vi "Send Dialog.vi"() -> ()   [LabVIEW 2011, in "CAN FD.lvlib"]
uses:
  CAN FD.lvlib
  Typedef/Send Data.ctl
  data_type/ZCAN_Transmit_Data.ctl
  data_type/ZCAN_TransmitFD_Data.ctl
panel:
  in  "Clear":bool
  in  "Data+":bool caption="数据递增"
  in  "ID+":bool caption="ID递增"
  in  "Stop":bool
  out "Count":u32 caption="发送统计" min=1 max=10000
  in  "Send":bool
  in  "spare":u32=100 caption="发送间隔(ms)" max=10000
  in  "Frames":u32=1 caption="单次帧数" min=1 max=1000
  in  "Times":i32=1 caption="发送次数(-1=持续)" min=-1
  in  "Data":string="01 23 45 67 89 AB CD EF" caption="数据输入"
  in  "Len":u8(ring)=8 caption="数据长度" items=["0"=0, "1"=1, "2"=2, "3"=3, "4"=4, "5"=5, "6"=6, "7"=7, "8"=8, "12"=12, "16"=16, "20"=20, "24"=24, "32"=32, "48"=48, "64"=64]
  in  "ID":u32=256 max=2047 format="0x%03x"
  in  "FD":u8(ring) caption="CANFD加速" items=["不加速", "加速"]
  in  "Protocol":u32(ring) caption="协议" items=["CAN", "CANFD"]
  in  "Type":u32(ring) caption="帧格式" items=["标准帧", "扩展帧"]
  in  "Format":u32(ring) caption="帧格式" items=["数据帧", "远程帧"]
  in  "Mode":u32(ring) caption="发送方式" items=["正常发送", "单次发送", "自发自收", "单次自发自收"]
  in  "Channel":u32(ring) caption="通道选择" items=["USBCANFD-200U 设备0 通道0"=2686976, "USBCANFD-200U 设备0 通道1"=2686977]
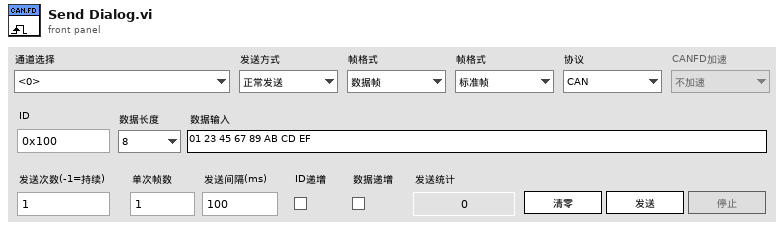
[diagram p1: front panel]
types:
  T1 = typedef "CAN FD.lvlib/Send Data.ctl" = cluster{"Handle":u32, "Frames":u32, "Spare":u32, "Times":i32, "ID+":bool, "Data+":bool, "Type":enum16{"CAN", "CANFD"}, "Data":variant}
  T2 = typedef "ZCAN_Transmit_Data.ctl" = cluster{"帧类型":u32, "帧格式":u32, "ID":u32, "数据长度":u8, "DATA":cluster{"CAN数据[0]":u8, "CAN数据[1]":u8, "CAN数据[2]":u8, "CAN数据[3]":u8, "CAN数据[4]":u8, "CAN数据[5]":u8, "CAN数据[6]":u8, "CAN数据[7]":u8}, "发送方式":u32}
  T3 = typedef "ZCAN_TransmitFD_Data.ctl" = cluster{"帧类型":u32, "帧格式":u32, "ID":u32, "数据长度":u8, "CANFD加速？":u8, "DATA":cluster{"CAN数据[0]":u8, "CAN数据[1]":u8, "CAN数据[2]":u8, "CAN数据[3]":u8, "CAN数据[4]":u8, "CAN数据[5]":u8, "CAN数据[6]":u8, "CAN数据[7]":u8, "CAN数据[8]":u8, "CAN数据[9]":u8, "CAN数据[10]":u8, "CAN数据[11] ":u8, "CAN数据[12] ":u8, "CAN数据[13] ":u8, "CAN数据[14] ":u8, "CAN数据[15] ":u8, "CAN数据[16]":u8, "CAN数据[17]":u8, "CAN数据[18]":u8, "CAN数据[19]":u8, "CAN数据[20]":u8, "CAN数据[21]":u8, "CAN数据[22]":u8, "CAN数据[23]":u8, "CAN数据[24] ":u8, "CAN数据[25]":u8, "CAN数据[26]":u8, "CAN数据[27]":u8, "CAN数据[28]":u8, "CAN数据[29]":u8, "CAN数据[30]":u8, "CAN数据[31]":u8, "CAN数据[32]":u8, "CAN数据[33]":u8, "CAN数据[34]":u8, "CAN数据[35]":u8, "CAN数据[36]":u8, "CAN数据[37]":u8, "CAN数据[38]":u8, "CAN数据[39]":u8, "CAN数据[40]":u8, "CAN数据[41]":u8, "CAN数据[42]":u8, "CAN数据[43]":u8, "CAN数据[44]":u8, "CAN数据[45]":u8, "CAN数据[46]":u8, "CAN数据[47]":u8, "CAN数据[48]":u8, "CAN数据[49]":u8, "CAN数据[50]":u8, "CAN数据[51]":u8, "CAN数据[52]":u8, "CAN数据[53]":u8, "CAN数据[54]":u8, "CAN数据[55]":u8, "CAN数据[56]":u8, "CAN数据[57]":u8, "CAN数据[58]":u8, "CAN数据[59]":u8, "CAN数据[60]":u8, "CAN数据[61]":u8, "CAN数据[62]":u8, "CAN数据[63]":u8}, "发送方式":u32}
  T4 = cluster{"Data[0]":u8, "Data[1]":u8, "Data[2]":u8, "Data[3]":u8, "Data[4]":u8, "Data[5]":u8, "Data[6]":u8, "Data[7]":u8}
  T5 = cluster{"Data[0]":u8, "Data[1]":u8, "Data[2]":u8, "Data[3]":u8, "Data[4]":u8, "Data[5]":u8, "Data[6]":u8, "Data[7]":u8, "Data[8]":u8, "Data[9]":u8, "Data[10]":u8, "Data[11]":u8, "Data[12]":u8, "Data[13]":u8, "Data[14]":u8, "Data[15]":u8, "Data[16]":u8, "Data[17]":u8, "Data[18]":u8, "Data[19]":u8, "Data[20]":u8, "Data[21]":u8, "Data[22]":u8, "Data[23]":u8, "Data[24]":u8, "Data[25]":u8, "Data[26]":u8, "Data[27]":u8, "Data[28]":u8, "Data[29]":u8, "Data[30]":u8, "Data[31]":u8, "Data[32]":u8, "Data[33]":u8, "Data[34]":u8, "Data[35]":u8, "Data[36]":u8, "Data[37]":u8, "Data[38]":u8, "Data[39]":u8, "Data[40]":u8, "Data[41]":u8, "Data[42]":u8, "Data[43]":u8, "Data[44]":u8, "Data[45]":u8, "Data[46]":u8, "Data[47]":u8, "Data[48]":u8, "Data[49]":u8, "Data[50]":u8, "Data[51]":u8, "Data[52]":u8, "Data[53]":u8, "Data[54]":u8, "Data[55]":u8, "Data[56]":u8, "Data[57]":u8, "Data[58]":u8, "Data[59]":u8, "Data[60]":u8, "Data[61]":u8, "Data[62]":u8, "Data[63]":u8}
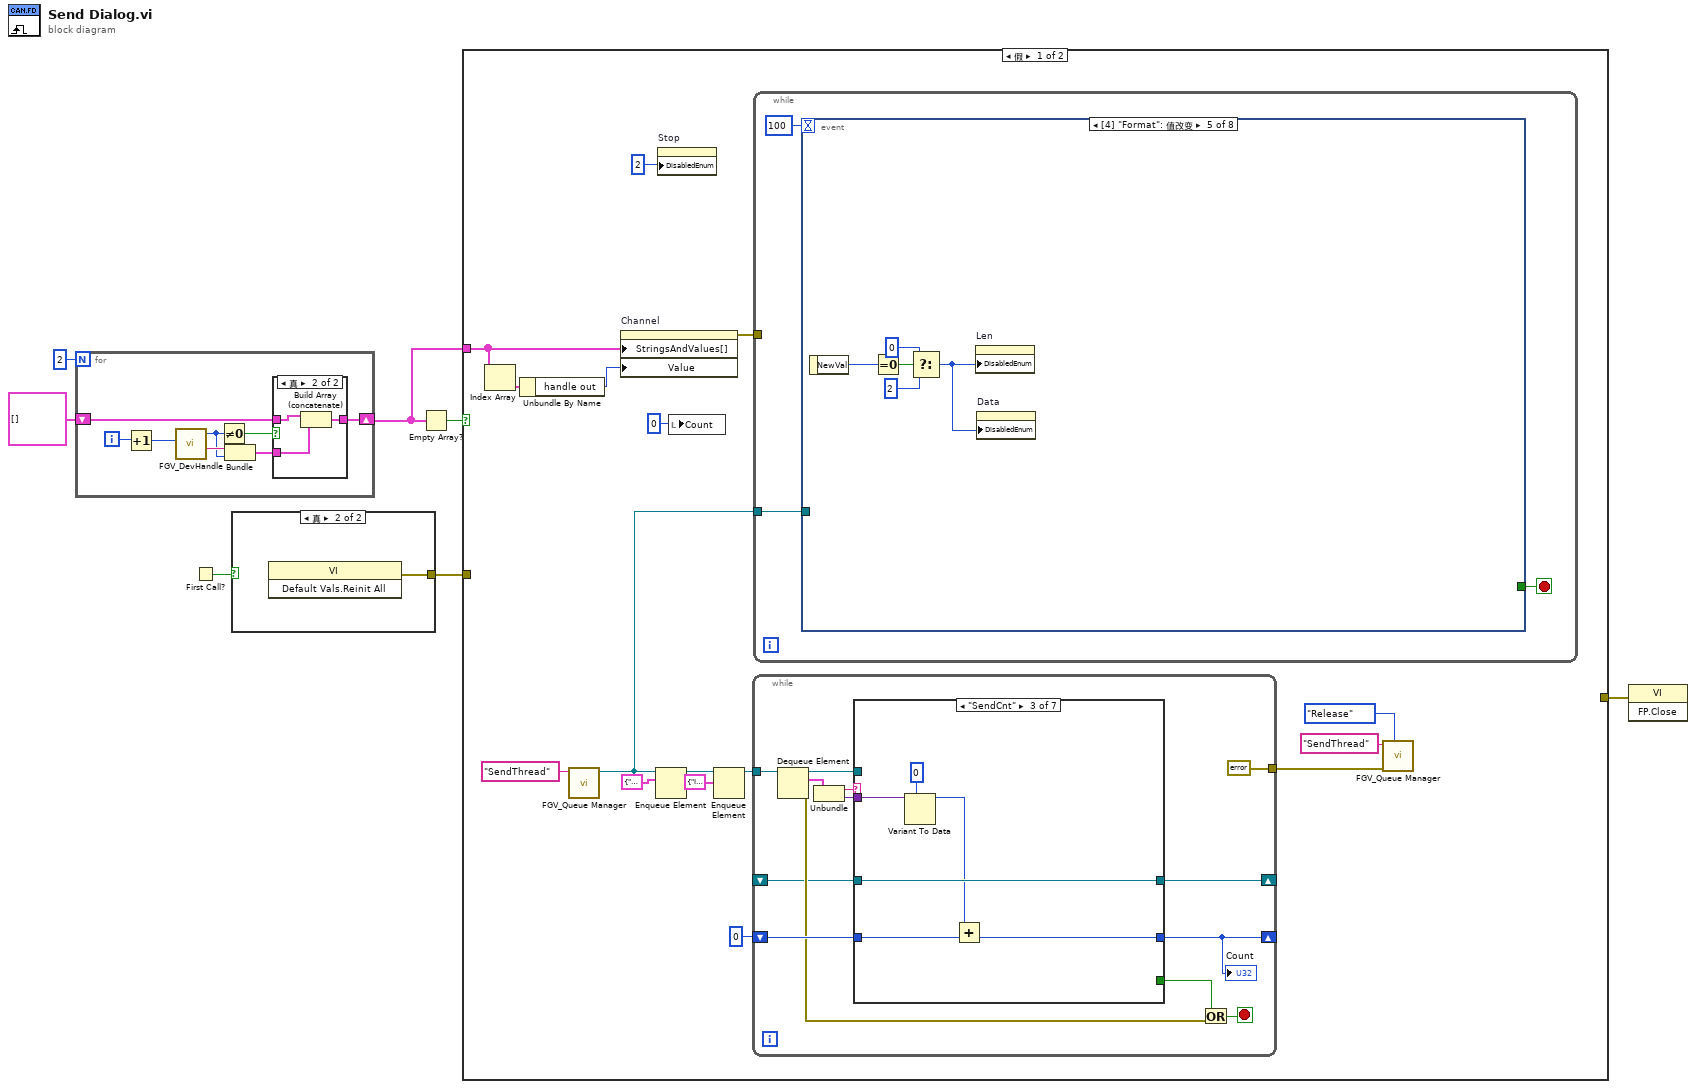
[diagram p0: block diagram]
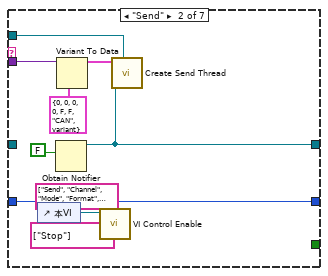
[diagram p4: hidden frame]
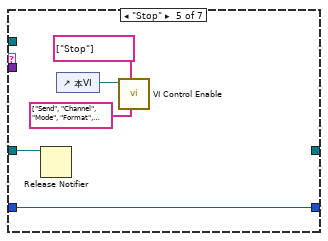
[diagram p6: hidden frame]
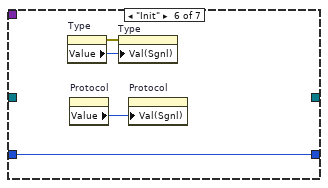
[diagram p7: hidden frame]
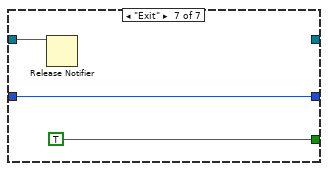
[diagram p8: hidden frame]
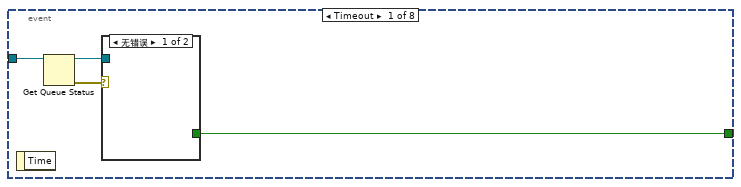
[diagram p9: hidden frame]
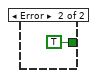
[diagram p10: hidden frame]
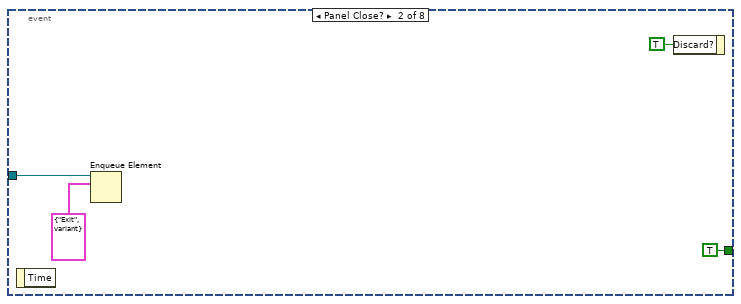
[diagram p11: hidden frame]
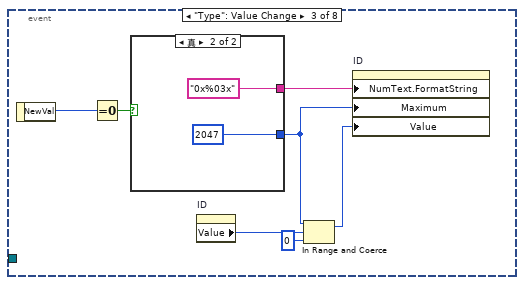
[diagram p12: hidden frame]
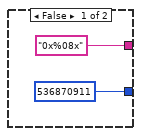
[diagram p13: hidden frame]
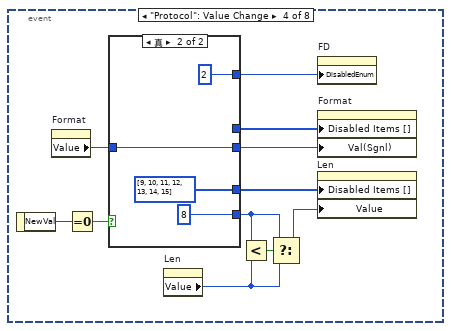
[diagram p14: hidden frame]
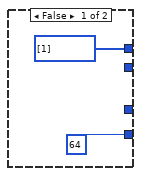
[diagram p15: hidden frame]
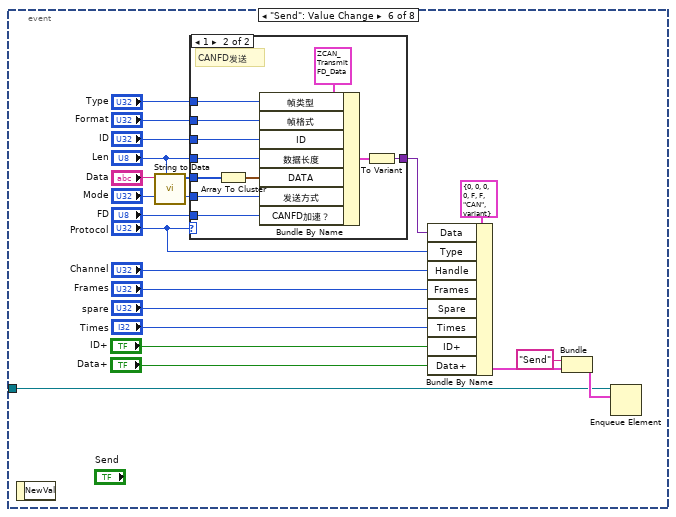
[diagram p16: hidden frame]
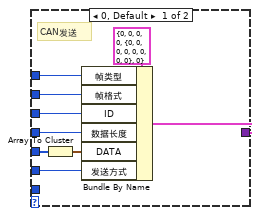
[diagram p17: hidden frame]
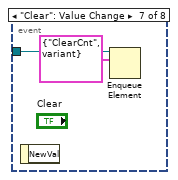
[diagram p18: hidden frame]
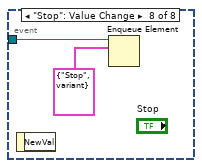
[diagram p19: hidden frame]
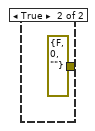
[diagram p20: hidden frame]
diagram:
  n1 = for {
    N: 2 -> [_]
    shift-right: [w9] -> w5
    shift-left: cluster{"Name out":string, "handle out":u32}[] [] -> [w8]
    i -> [w15]
    n2 = Increment(x=w15) -> (x+1=w14:i32)
    n3 = call "FGV_DevHandle.vi"("Type"=w14) -> ("Name out"=w13:string, "handle out"=w12:u32)  [unwired: 8 in, 1 out]
    n4 = Not Equal To 0?(x=w12) -> (x != 0?=w11:bool)
    n5 = Bundle("Name out"=w13, "handle out"=w12) -> (w10:cluster{"Name out":string, "handle out":u32})  [unwired: 1 in]
    n6 = case shown="真" w11 {
      tunnel: w10 -> [_ w19]
      tunnel: [w16 w18] -> w9
      tunnel: w8 -> [w16 w17]
      frame False {
      }
      frame True {
        n7 = Build Array (concatenate)(w17, w19) -> (w18:cluster{"Name out":string, "handle out":u32}[])
      }
    }
  }
  n8 = First Call?() -> (First Call?: T/F=w3:bool)
  n9 = case shown="真" w3 {
    tunnel: [_ w20] -> w2
    frame False {
    }
    frame True {
      n10 = invoke class="VI" method="Default Vals.Reinit All"() -> (error out=w20:errorcluster)  [unwired: 3 in, 2 out]
    }
  }
  n11 = Empty Array?(array=w5) -> (empty?=w4:bool)
  n12 = case shown="假" w4 {
    tunnel: w5 -> [w36 _]
    tunnel: w2 -> [_ _]
    tunnel: [_ errorcluster {"status"=FALSE, "code"=0, "source"=""} ("error constant")] -> w1
    frame False {
      n13 = Index Array(array=w36) -> (element=w35:cluster{"Name out":string, "handle out":u32})  [unwired: 1 in]
      n14 = Unbundle By Name(w35) -> ("handle out"=w34:u32)
      n15 = call "FGV_Queue Manager.vi"("Name"="SendThread") -> ("Queue"=w27:refnum<queue>)  [unwired: 8 in, 2 out]
      n16 = property on="Channel" class="Ring (严格)"("StringsAndValues[]"=w36, "Value"=w34) -> (error out=w33:errorcluster)  [unwired: 2 in, 1 out]
      n17 = Enqueue Element(queue=w27, element=cluster{"ID":string, "Data":variant} {"ID"="Stop", "Data"=variant} ("元素")) -> (queue out=w23:refnum<queue>)  [unwired: 2 in, 2 out]
      n18 = property on="Stop" class="Bool"("DisabledEnum"=2) -> ()  [unwired: 2 in, 2 out]
      n19 = local write "Count"(u32 0 ("Count")) -> ()
      n20 = Enqueue Element(queue=w23, element=cluster{"ID":string, "Data":variant} {"ID"="Init", "Data"=variant} ("元素")) -> (queue out=w22:refnum<queue>)  [unwired: 2 in, 2 out]
      n21 = while {
        tunnel: w22 -> [w49]
        shift-right: [w44] -> _
        shift-left: u32 0 -> [w45]
        tunnel: [errorcluster {"status"=FALSE, "code"=0, "source"=""} ("error constant")] -> w26
        shift-right: [w38] -> _
        shift-left: _ -> [w37]
        stop <- w39 stop-if-true
        n22 = Dequeue Element(queue=w49) -> (queue out=w43:refnum<queue>, element=w48:cluster{"ID":string, "Data":variant}, error out=w40:errorcluster)  [unwired: 2 in, 1 out]
        n23 = Unbundle(w48) -> ("ID"=w47:string, "Data"=w46:variant)
        n24 = case shown="\"SendCnt\"" w47 {
          tunnel: w46 -> [_ w60 w65 _ _ _ _]
          tunnel: [_ _ _ _ _ _ TRUE] -> w41
          tunnel: w45 -> [w50 w51 w63 _ w72 w76 w78]
          tunnel: [w50 w51 w61 _ w72 w76 w78] -> w44
          tunnel: w43 -> [_ w56 _ _ _ _ _]
          tunnel: [_ w55 w66 w67 _ _ _] -> w38
          tunnel: w37 -> [_ _ w66 w67 w68 _ w77]
          frame Default {
          }
          frame "Send" {
            n25 = control-ref of="本VI"() -> (w52:refnum<vi>)
            n26 = Obtain Notifier(notification data type=FALSE) -> (notifier out=w55:refnum<notifier>)  [unwired: 3 in, 2 out]
            n27 = Variant To Data(type=T1 {"Handle"=0, "Frames"=0, "Spare"=0, "Times"=0, "ID+"=FALSE, "Data+"=FALSE, "Type"=enum."CAN", "Data"=variant} ("Send Data"), Variant=w60) -> (data=w57:T1)  [unwired: 1 in, 1 out]
            n28 = call "VI Control Enable.vi"("Enable List"=string[] ["Stop"], "Disable List"=string[] ["Send", "Channel", "Mode", "Format", "Type", "Protocol", "FD", "ID", "Len", "Data", "Times", "Frames", "spare", "ID+", "Data+"], "VI引用句柄"=w52) -> ()  [unwired: 9 in]
            n29 = call "Create Send Thread.vi"("SendQueue"=w56, "StopNotifier"=w55, "Send Data"=w57) -> ()  [unwired: 9 in]
          }
          frame "SendCnt" {
            n30 = Variant To Data(type=u32 0, Variant=w65) -> (data=w62:u32)  [unwired: 1 in, 1 out]
            n31 = Add(x=w62, y=w63) -> (x+y=w61:u32)
          }
          frame "ClearCnt" {
          }
          frame "Stop" {
            n32 = Release Notifier(notifier=w68) -> ()  [unwired: 2 in, 3 out]
            n33 = control-ref of="本VI"() -> (w71:refnum<vi>)
            n34 = call "VI Control Enable.vi"("Enable List"=string[] ["Send", "Channel", "Mode", "Format", "Type", "Protocol", "FD", "ID", "Len", "Data", "Times", "Frames", "spare", "ID+", "Data+"] ("Disable List"), "Disable List"=string[] ["Stop"] ("Enable List"), "VI引用句柄"=w71) -> ()  [unwired: 9 in]
          }
          frame "Init" {
            n35 = property on="Type" class="Ring (严格)"() -> (error out=w74:errorcluster, "Value"=w73:u32)  [unwired: 2 in, 1 out]
            n36 = property on="Protocol" class="Ring (严格)"() -> ("Value"=w75:u32)  [unwired: 2 in, 2 out]
            n37 = property on="Type" class="Ring (严格)"(error in=w74, "Val(Sgnl)"=w73) -> ()  [unwired: 1 in, 2 out]
            n38 = property on="Protocol" class="Ring (严格)"("Val(Sgnl)"=w75) -> ()  [unwired: 2 in, 2 out]
          }
          frame "Exit" {
            n39 = Release Notifier(notifier=w77) -> ()  [unwired: 2 in, 3 out]
          }
        }
        "Count" <- w44
        n40 = Or(x=w41, y=w40) -> (x .or. y?=w39:bool)
      }
      n41 = while {
        tunnel: w33 -> [_]
        tunnel: w27 -> [w81]
        stop <- w82 stop-if-true
        n42 = event shown="[4] \"Format\": 值改变" {
          selector: _ -> [_ _ _ _ _ _ _ _]
          dyn-events: _ -> [_ _ _ _ _ _ _ _]
          timeout: 100 -> [_ _ _ _ _ _ _ _]
          tunnel: [w84 TRUE _ _ _ _ _ _] -> w82
          tunnel: w81 -> [w86 w90 _ _ _ w132 w167 w169]
          event Timeout {
            n43 = event-data() -> ()  [unwired: 1 in, 1 out]
            n44 = Get Queue Status(queue=w86) -> (queue out=w83:refnum<queue>, error out=w85:errorcluster)  [unwired: 2 in, 6 out]
            n45 = case shown="无错误" w85 {
              tunnel: [_ TRUE] -> w84
              tunnel: w83 -> [_ _]
              frame No Error {
              }
              frame Error {
              }
            }
          }
          event Panel Close? {
            n46 = event-data() -> ()  [unwired: 1 in, 1 out]
            n47 = Enqueue Element(queue=w90, element=cluster{"ID":string, "Data":variant} {"ID"="Exit", "Data"=variant} ("元素")) -> ()  [unwired: 2 in, 3 out]
            n48 = event-data("Discard?"=TRUE ("放弃？")) -> ()  [unwired: 1 in, 1 out]
          }
          event "Type": Value Change {
            n49 = event-data() -> ("NewVal"=w98:u32)  [unwired: 1 in]
            n50 = Equal To 0?(x=w98) -> (x = 0?=w97:bool)
            n51 = case shown="真" w97 {
              tunnel: ["0x%08x" "0x%03x"] -> w96
              tunnel: [u32 536870911 u32 2047] -> w93
              frame False {
              }
              frame True {
              }
            }
            n52 = property on="ID" class="DigNum (严格)"() -> ("Value"=w95:u32)  [unwired: 2 in, 2 out]
            n53 = In Range and Coerce(upper limit=w93, x=w95, lower limit=u32 0 ("下限")) -> (coerced(x)=w92:u32)  [unwired: 1 out]
            n54 = property on="ID" class="DigNum (严格)"("NumText.FormatString"=w96, "Maximum"=w93, "Value"=w92) -> ()  [unwired: 2 in, 2 out]
          }
          event "Protocol": Value Change {
            n55 = event-data() -> ("NewVal"=w113:u32)  [unwired: 1 in]
            n56 = property on="Format" class="Ring (严格)"() -> ("Value"=w104:u32)  [unwired: 2 in, 2 out]
            n57 = Equal To 0?(x=w113) -> (x = 0?=w112:bool)
            n58 = case shown="真" w112 {
              tunnel: [_ i32[] [9, 10, 11, 12, 13, 14, 15] ("禁用项[]")] -> w111
              tunnel: [u8 64 u8 8] -> w109
              tunnel: [i32[] [1] ("禁用项[]") _] -> w106
              tunnel: [_ w117] -> w105
              tunnel: w104 -> [_ w117]
              tunnel: [_ 2] -> w103
              frame False {
              }
              frame True {
              }
            }
            n59 = property on="Len" class="Ring (严格)"() -> ("Value"=w108:u8)  [unwired: 2 in, 2 out]
            n60 = Less?(x=w109, y=w108) -> (x < y?=w110:bool)
            n61 = Select(t=w109, s=w110, f=w108) -> (s? t:f=w107:u8)
            n62 = property on="FD" class="Ring (严格)"("DisabledEnum"=w103) -> ()  [unwired: 2 in, 2 out]
            n63 = property on="Format" class="Ring (严格)"("Disabled Items []"=w106, "Val(Sgnl)"=w105) -> ()  [unwired: 2 in, 2 out]
            n64 = property on="Len" class="Ring (严格)"("Disabled Items []"=w111, "Value"=w107) -> ()  [unwired: 2 in, 2 out]
          }
          event "Format": Value Change {
            n65 = event-data() -> ("NewVal"=w121:u32)  [unwired: 1 in]
            n66 = Equal To 0?(x=w121) -> (x = 0?=w124:bool)
            n67 = Select(t=0, s=w124, f=2) -> (s? t:f=w120:i32)
            n68 = property on="Len" class="Ring (严格)"("DisabledEnum"=w120) -> ()  [unwired: 2 in, 2 out]
            n69 = property on="Data" class="Str"("DisabledEnum"=w120) -> ()  [unwired: 2 in, 2 out]
          }
          event "Send": Value Change {
            n70 = event-data() -> ()  [unwired: 1 in, 1 out]
            n71 = call "String to Data.vi"("Len"="Len", "String"="Data") -> ("Data"=w140:u8[])  [unwired: 8 in, 1 out]
            n72 = case shown="1" "Protocol" {
              tunnel: "Type" -> [w153 w165]
              tunnel: "Format" -> [w152 w164]
              tunnel: "ID" -> [w151 w163]
              tunnel: "Len" -> [w150 w162]
              tunnel: w140 -> [w149 w161]
              tunnel: "Mode" -> [w147 w159]
              tunnel: "FD" -> [_ w157]
              tunnel: [w146 w155] -> w130
              frame 0, Default {
                # "CAN发送"
                n73 = Array To Cluster(array=w149) -> (cluster=w148:T4)
                n74 = Bundle By Name(cluster=T2 {"帧类型"=0, "帧格式"=0, "ID"=0, "数据长度"=0, "DATA"={"CAN数据[0]"=0, "CAN数据[1]"=0, "CAN数据[2]"=0, "CAN数据[3]"=0, "CAN数据[4]"=0, "CAN数据[5]"=0, "CAN数据[6]"=0, "CAN数据[7]"=0}, "发送方式"=0} ("ZCAN_Transmit_Data"), "帧类型"=w153, "帧格式"=w152, "ID"=w151, "数据长度"=w150, "DATA"=w148, "发送方式"=w147) -> (w146:T2)
              }
              frame 1 {
                # "CANFD发送"
                n75 = Array To Cluster(array=w161) -> (cluster=w160:T5)
                n76 = Bundle By Name(cluster=T3 {"帧类型"=0, "帧格式"=0, "ID"=0, "数据长度"=0, "CANFD加速？"=0, "DATA"={"CAN数据[0]"=0, "CAN数据[1]"=0, "CAN数据[2]"=0, "CAN数据[3]"=0, "CAN数据[4]"=0, "CAN数据[5]"=0, "CAN数据[6]"=0, "CAN数据[7]"=0, "CAN数据[8]"=0, "CAN数据[9]"=0, "CAN数据[10]"=0, "CAN数据[11] "=0, "CAN数据[12] "=0, "CAN数据[13] "=0, "CAN数据[14] "=0, "CAN数据[15] "=0, "CAN数据[16]"=0, "CAN数据[17]"=0, "CAN数据[18]"=0, "CAN数据[19]"=0, "CAN数据[20]"=0, "CAN数据[21]"=0, "CAN数据[22]"=0, "CAN数据[23]"=0, "CAN数据[24] "=0, "CAN数据[25]"=0, "CAN数据[26]"=0, "CAN数据[27]"=0, "CAN数据[28]"=0, "CAN数据[29]"=0, "CAN数据[30]"=0, "CAN数据[31]"=0, "CAN数据[32]"=0, "CAN数据[33]"=0, "CAN数据[34]"=0, "CAN数据[35]"=0, "CAN数据[36]"=0, "CAN数据[37]"=0, "CAN数据[38]"=0, "CAN数据[39]"=0, "CAN数据[40]"=0, "CAN数据[41]"=0, "CAN数据[42]"=0, "CAN数据[43]"=0, "CAN数据[44]"=0, "CAN数据[45]"=0, "CAN数据[46]"=0, "CAN数据[47]"=0, "CAN数据[48]"=0, "CAN数据[49]"=0, "CAN数据[50]"=0, "CAN数据[51]"=0, "CAN数据[52]"=0, "CAN数据[53]"=0, "CAN数据[54]"=0, "CAN数据[55]"=0, "CAN数据[56]"=0, "CAN数据[57]"=0, "CAN数据[58]"=0, "CAN数据[59]"=0, "CAN数据[60]"=0, "CAN数据[61]"=0, "CAN数据[62]"=0, "CAN数据[63]"=0}, "发送方式"=0} ("ZCAN_TransmitFD_Data"), "帧类型"=w165, "帧格式"=w164, "ID"=w163, "数据长度"=w162, "DATA"=w160, "发送方式"=w159, "CANFD加速？"=w157) -> (w156:T3)
                n77 = To Variant(anything=w156) -> (Variant=w155:variant)
              }
            }
            n78 = Bundle By Name(cluster=T1 {"Handle"=0, "Frames"=0, "Spare"=0, "Times"=0, "ID+"=FALSE, "Data+"=FALSE, "Type"=enum."CAN", "Data"=variant} ("Send Data"), "Data"=w130, "Type"="Protocol", "Handle"="Channel", "Frames"="Frames", "Spare"="spare", "Times"="Times", "ID+"="ID+", "Data+"="Data+") -> (w134:T1)
            n79 = Bundle("Send", "Send Data"=w134) -> (w136:cluster{string, "Send Data":T1})  [unwired: 1 in]
            n80 = Enqueue Element(queue=w132, element=w136) -> ()  [unwired: 2 in, 3 out]
          }
          event "Clear": Value Change {
            n81 = event-data() -> ()  [unwired: 1 in, 1 out]
            n82 = Enqueue Element(queue=w167, element=cluster{"ID":string, "Data":variant} {"ID"="ClearCnt", "Data"=variant} ("元素")) -> ()  [unwired: 2 in, 3 out]
          }
          event "Stop": Value Change {
            n83 = event-data() -> ()  [unwired: 1 in, 1 out]
            n84 = Enqueue Element(queue=w169, element=cluster{"ID":string, "Data":variant} {"ID"="Stop", "Data"=variant} ("元素")) -> ()  [unwired: 2 in, 3 out]
          }
        }
      }
      n85 = call "FGV_Queue Manager.vi"("Methods"=enum16{"Init", "Get", "Release", "Destroy"}."Release", "error in (no error)"=w26, "Name"="SendThread") -> ()  [unwired: 6 in, 3 out]
    }
    frame True {
    }
  }
  n86 = invoke class="VI" method="FP.Close"(error in=w1) -> ()  [unwired: 2 in, 3 out]
